vi "performance data.vi"(11 "CPU %":sgl) -> (0 "Dash IPS":u32, 1 "Dash mSPI":u32, 2 "Main IPS":u32, 3 "Main mSPI":u32, 5 "Stats":sgl[][](graph))   [LabVIEW 2014]
uses:
  <vilib>/Rock Robotics/Network Tables/NT Read Numeric Array.vi
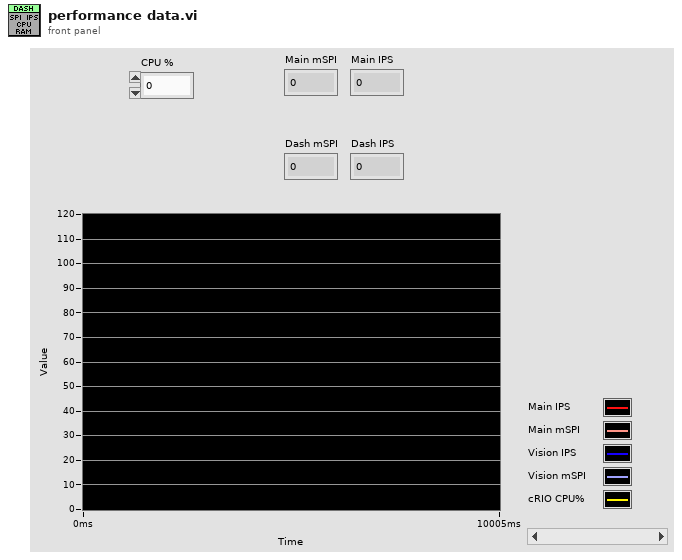
[diagram p1: front panel]
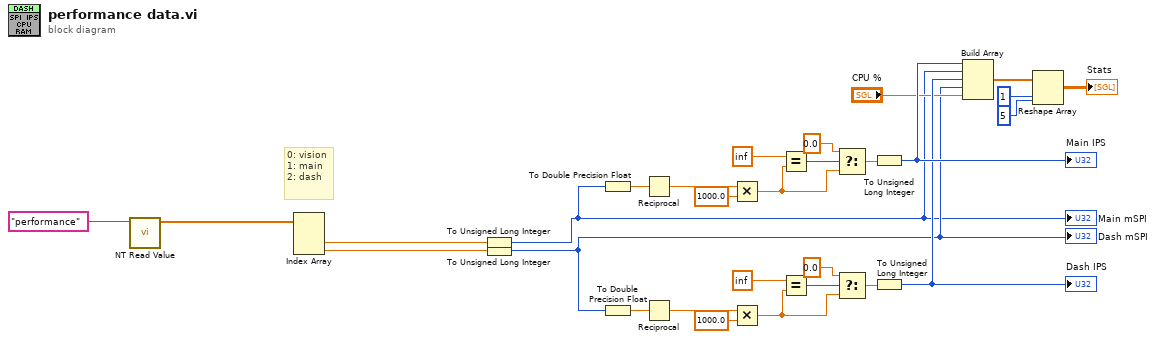
[diagram p0: block diagram]
diagram:
  # "0: vision\n1: main\n2: dash"
  n1 = call-poly <vilib>:"NT Read Value.vi"("Name"="performance") -> ("Numeric Array"=w9:dbl[])  [unwired: 9 in, 1 out]
  n2 = Index Array(array=w9) -> (element #2=w7:dbl, element #3=w8:dbl)  [unwired: 3 in, 1 out]
  n3 = To Unsigned Long Integer(number=w7) -> (unsigned 32bit integer=w5:u32)
  "Main mSPI" <- w5
  n4 = To Unsigned Long Integer(number=w8) -> (unsigned 32bit integer=w6:u32)
  "Dash mSPI" <- w6
  n5 = To Double Precision Float(number=w5) -> (double precision float=w27:dbl)
  n6 = To Double Precision Float(number=w6) -> (double precision float=w20:dbl)
  n7 = Reciprocal(x=w27) -> (1/x=w28:dbl)
  n8 = Reciprocal(x=w20) -> (1/x=w19:dbl)
  n9 = Multiply(x=w28, y=1000.0) -> (x*y=w12:dbl)
  n10 = Multiply(x=w19, y=1000.0) -> (x*y=w11:dbl)
  n11 = Equal?(x=inf, y=w12) -> (x = y?=w26:bool)
  n12 = Equal?(x=inf, y=w11) -> (x = y?=w21:bool)
  n13 = Select(t=0.0, s=w26, f=w12) -> (s? t:f=w17:dbl)
  n14 = Select(t=0.0, s=w21, f=w11) -> (s? t:f=w16:dbl)
  n15 = To Unsigned Long Integer(number=w17) -> (unsigned 32bit integer=w15:u32)
  "Main IPS" <- w15
  n16 = To Unsigned Long Integer(number=w16) -> (unsigned 32bit integer=w14:u32)
  "Dash IPS" <- w14
  n17 = Build Array(w15, w5, w14, w6, "CPU %") -> (w2:sgl[])
  n18 = Reshape Array(w2, 1 ("dimension size"), 5 ("dimension size")) -> (→"Stats":sgl[][])
